vi "Configure Channel.vi"(0 "VISA resource name":refnum<visa-resource-name>, 1 "Enable Channel (T:Enable)":bool=TRUE, 2 "Enable Invert  (F: Disable)":bool, 5 "Channel (1: Channel 1)":u16(ring)=1 items=["Channel 1"=1, "Channel 2"=2, "Channel 3"=3, "Channel 4"=4], 7 "Vertical Coupling (1: DC)":u16(ring)=1 items=["AC", "DC", "Ground"], 9 "Probe Attenuation (3: 1X)":u16(ring)=3 items=["0.001X", "0.01X", "0.1X", "1X", "10X", "100X", "1000X"], 11 "error in (no error)":errorcluster, 12 "Vertical Range (10.0 V)":dbl=10.0, 13 "Vertical Offset (0.0 V)":dbl, 14 "Max Input Frequency (0.0 Hz)":dbl) -> (4 "VISA resource name out":refnum<visa-resource-name>, 15 "error out":errorcluster)   [LabVIEW 2011, in "Agilent DSO1000 Series.lvlib"]
doc: "Configures the common properties of the vertical subsystem of the oscilloscope for the specified channel. The properties include vertical coupling, vertical range, vertical offset, probe attenuation. Call this VI for each channel you want to enable to acquire waveforms.\n\n<B>Note:</B>\nThe channel settings will not be applied if the channel is not enabled."
uses:
  <instrlib>/Agilent DSO1000 Series/Agilent DSO1000 Series.lvlib
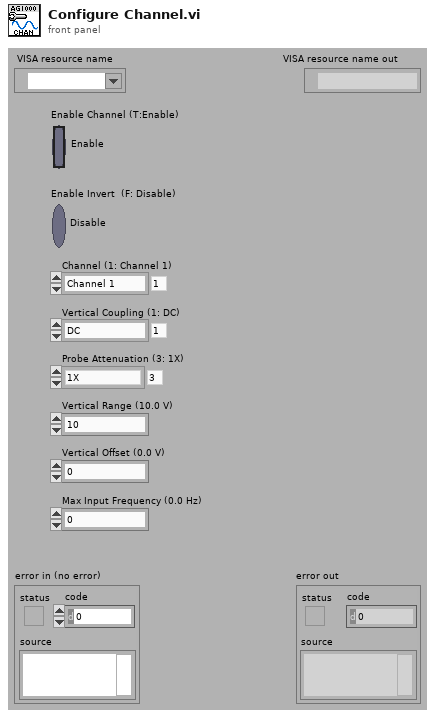
[diagram p1: front panel]
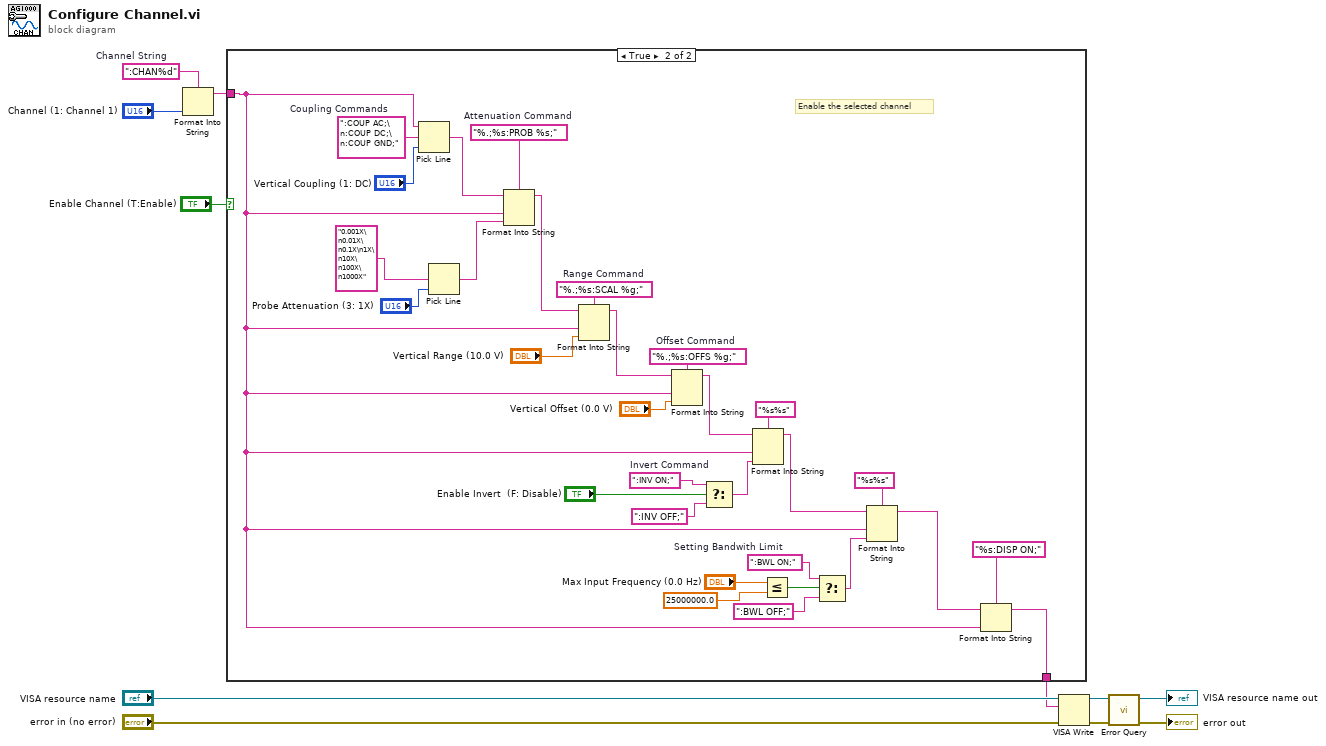
[diagram p0: block diagram]
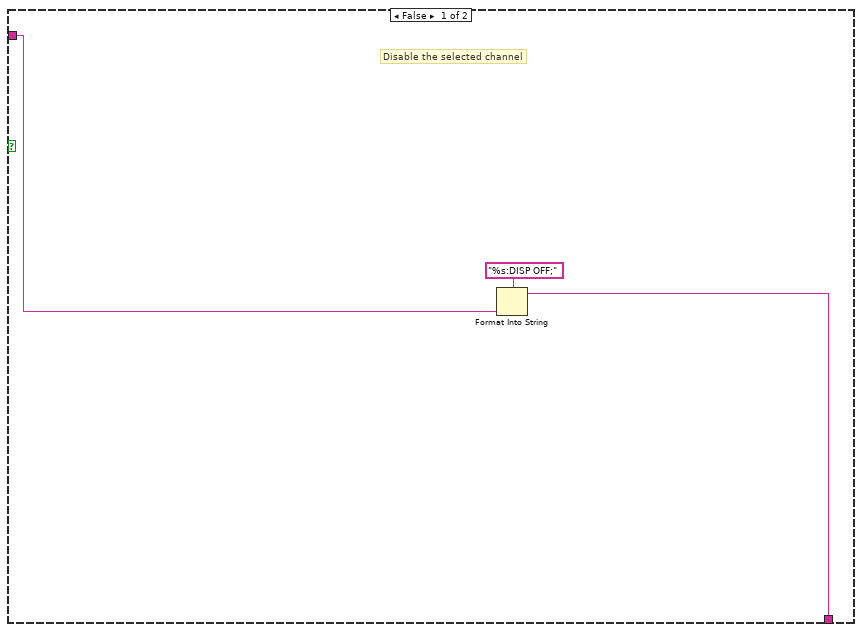
[diagram p2: hidden frame]
diagram:
  w3 = ":CHAN%d"  # Channel String
  n1 = Format Into String(format string=w3, "Channel (1: Channel 1)") -> (resulting string=w1:string)  [unwired: 2 in, 1 out]
  n2 = case shown="True" "Enable Channel (T:Enable)" {
    tunnel: [w13 w30] -> w5
    tunnel: w1 -> [w12 w17]
    frame False {
      # "Disable the selected channel"
      n3 = Format Into String(format string="%s:DISP OFF;", w12) -> (resulting string=w13:string)  [unwired: 2 in, 1 out]
    }
    frame True {
      w32 = ":BWL ON;"  # Setting Bandwith Limit
      w37 = ":INV ON;"  # Invert Command
      w20 = "%.;%s:PROB %s;"  # Attenuation Command
      w41 = "%.;%s:SCAL %g;"  # Range Command
      w43 = "%.;%s:OFFS %g;"  # Offset Command
      w45 = ":COUP AC;\n:COUP DC;\n:COUP GND;"  # Coupling Commands
      # "Enable the selected channel"
      n4 = Pick Line(string ("")=w17, multi-line string=w45, line index="Vertical Coupling (1: DC)") -> (output string=w19:string)
      n5 = Pick Line(multi-line string="0.001X\n0.01X\n0.1X\n1X\n10X\n100X\n1000X", line index="Probe Attenuation (3: 1X)") -> (output string=w21:string)  [unwired: 1 in]
      n6 = Format Into String(format string=w20, initial string=w19, w17, w21) -> (resulting string=w18:string)  [unwired: 1 in, 1 out]
      n7 = Format Into String(format string=w41, initial string=w18, w17, "Vertical Range (10.0 V)") -> (resulting string=w16:string)  [unwired: 1 in, 1 out]
      n8 = Format Into String(format string=w43, initial string=w16, w17, "Vertical Offset (0.0 V)") -> (resulting string=w15:string)  [unwired: 1 in, 1 out]
      n9 = Select(t=w37, s="Enable Invert  (F: Disable)", f=":INV OFF;") -> (s? t:f=w29:string)
      n10 = Format Into String(format string="%s%s", initial string=w15, w17, w29) -> (resulting string=w25:string)  [unwired: 1 in, 1 out]
      n11 = Less Or Equal?(x="Max Input Frequency (0.0 Hz)", y=25000000.0) -> (x <= y?=w33:bool)
      n12 = Select(t=w32, s=w33, f=":BWL OFF;") -> (s? t:f=w28:string)
      n13 = Format Into String(format string="%s%s", initial string=w25, w17, w28) -> (resulting string=w26:string)  [unwired: 1 in, 1 out]
      n14 = Format Into String(format string="%s:DISP ON;", initial string=w26, w17) -> (resulting string=w30:string)  [unwired: 1 in, 1 out]
    }
  }
  n15 = VISA Write(VISA resource name="VISA resource name", write buffer=w5, error in (no error)="error in (no error)") -> (VISA resource name out=w7:refnum<visa-resource-name>, error out=w6:errorcluster)  [unwired: 1 out]
  n16 = call <instrlib>:"Error Query.vi"("error in (no error)"=w6, "VISA resource name"=w7) -> ("error out"=→"error out":errorcluster, "VISA resource name out"=→"VISA resource name out":refnum<visa-resource-name>)  [unwired: 6 in, 2 out]
